vi "Accurate Measure With Setting - 複製 (2).vi"(0 "DMM ref in":refnum<visa-resource-name>, 1 "channel_count":i32=11, 2 "P_current_count":i32, 3 "N_current_count":i32, 5 "DMM error in":errorcluster, 7 "Accurate Measure Setting":T1, 9 "ESP32 ref in":refnum<visa-resource-name>, 11 "ESP32 error in":errorcluster, 12 "current_mode":u8[](array[numeric])=[0, 0, 0, 0, 0, 0, 0, 0, 0, 0, 0]) -> (4 "DMM ref out":refnum<visa-resource-name>, 6 "DMM error out":errorcluster, 8 "Accurate Data":dbl[](array[numeric]), 10 "ESP32 ref out":refnum<visa-resource-name>, 13 "time_out_count":i32, 14 "Standard Deviation of Data":dbl[](array[numeric]), 15 "ESP32 error out":errorcluster)   [LabVIEW 2023]
uses:
  <instrlib>/Agilent 3446X Series/Agilent 3446X Series.lvlib
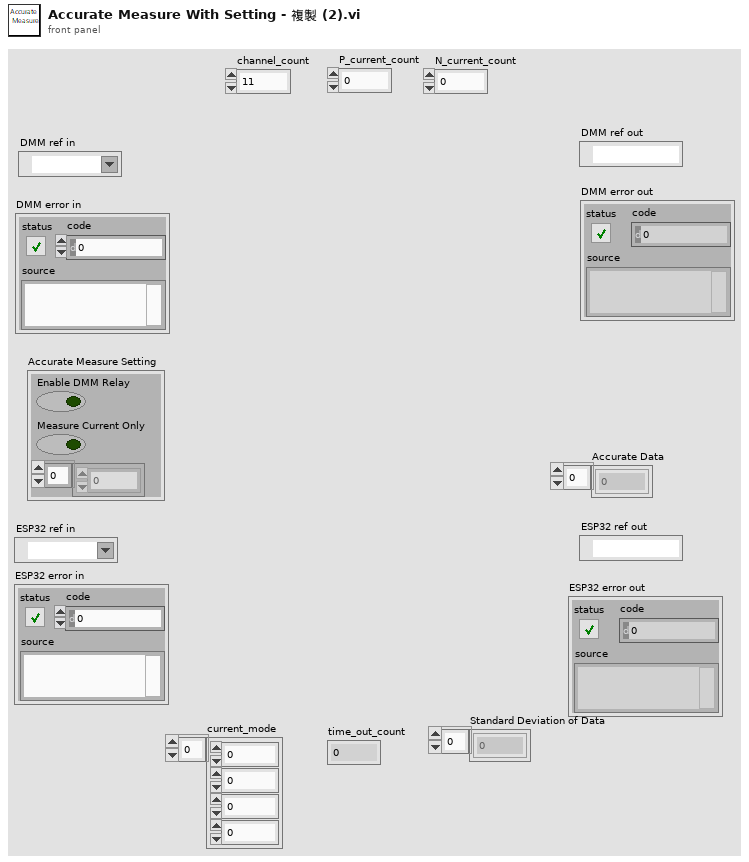
[diagram p1: front panel]
types:
  T1 = cluster{"Enable DMM Relay":bool, "Measure Current Only":bool, dbl[]}
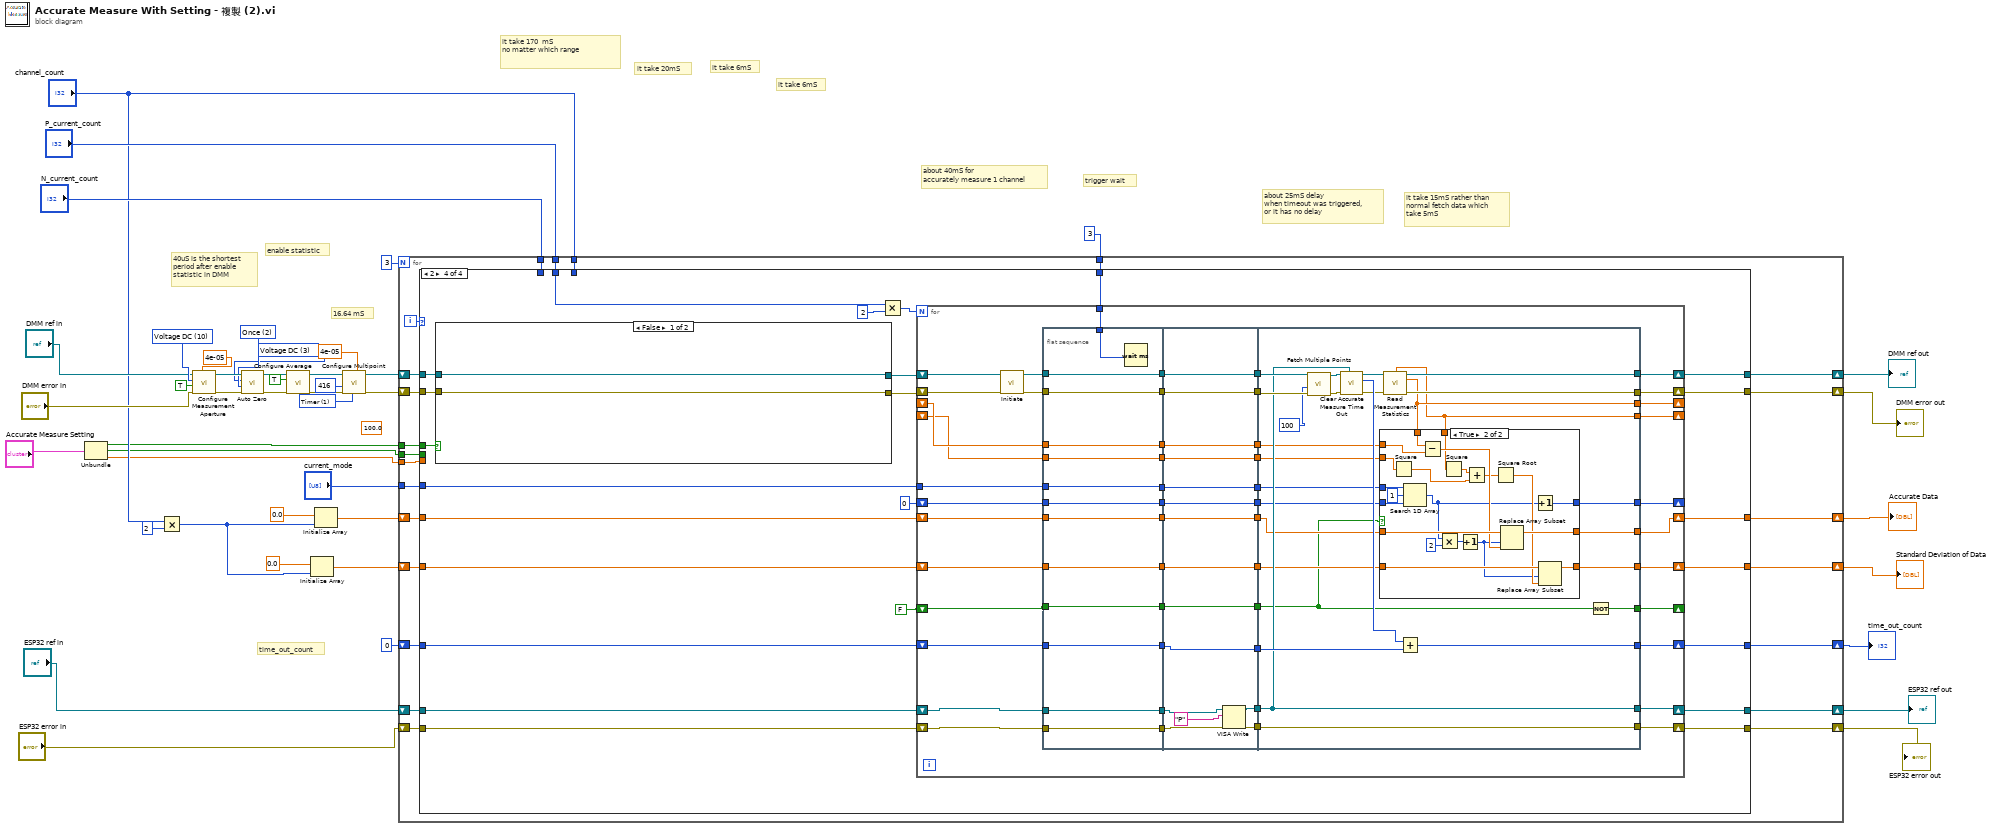
[diagram p0: block diagram]
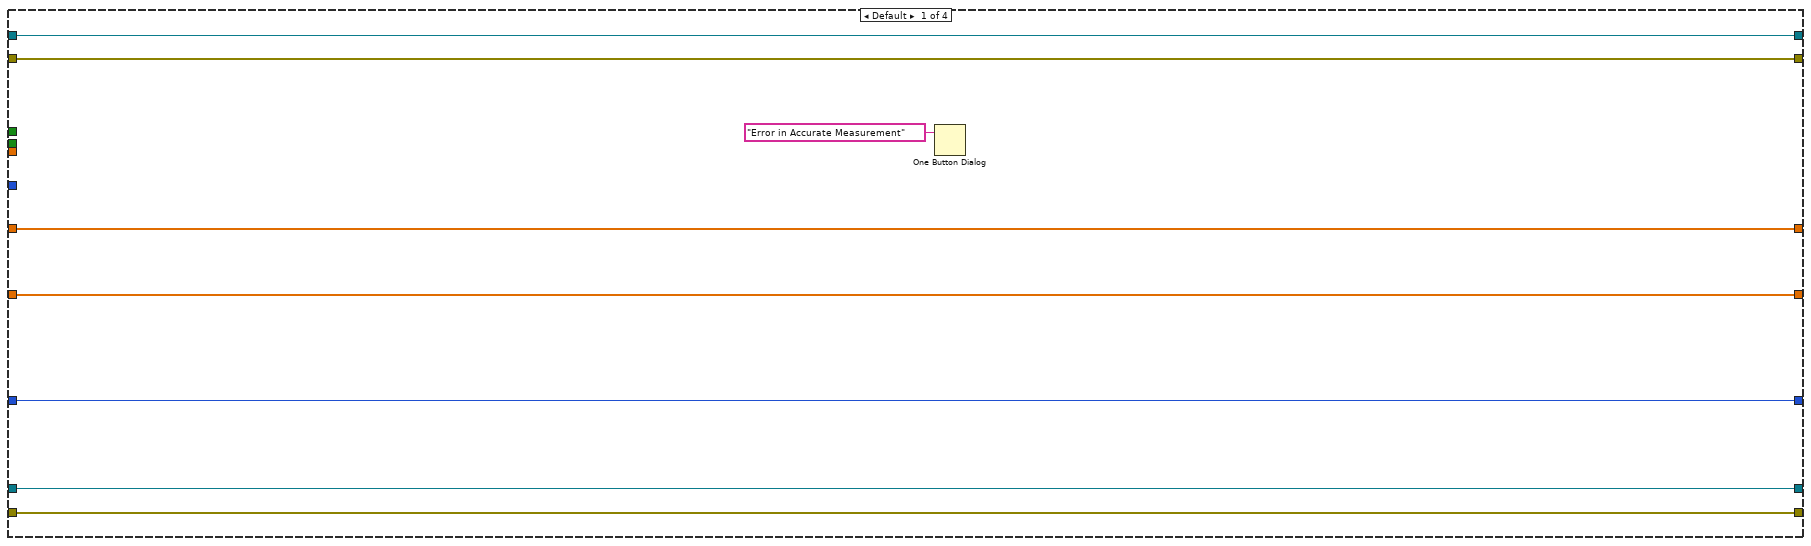
[diagram p2: hidden frame]
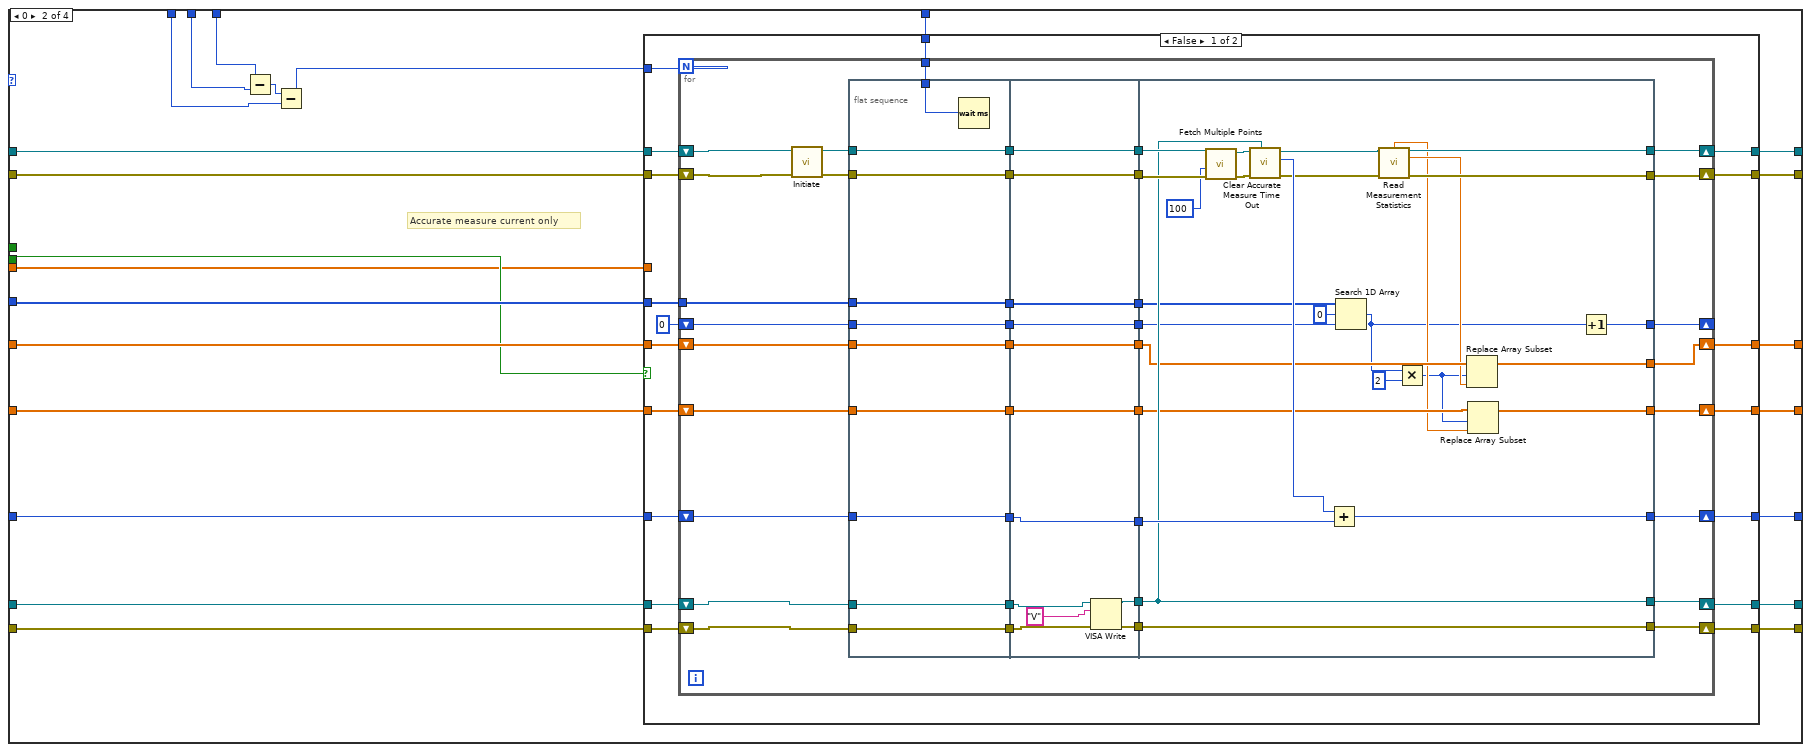
[diagram p3: hidden frame]
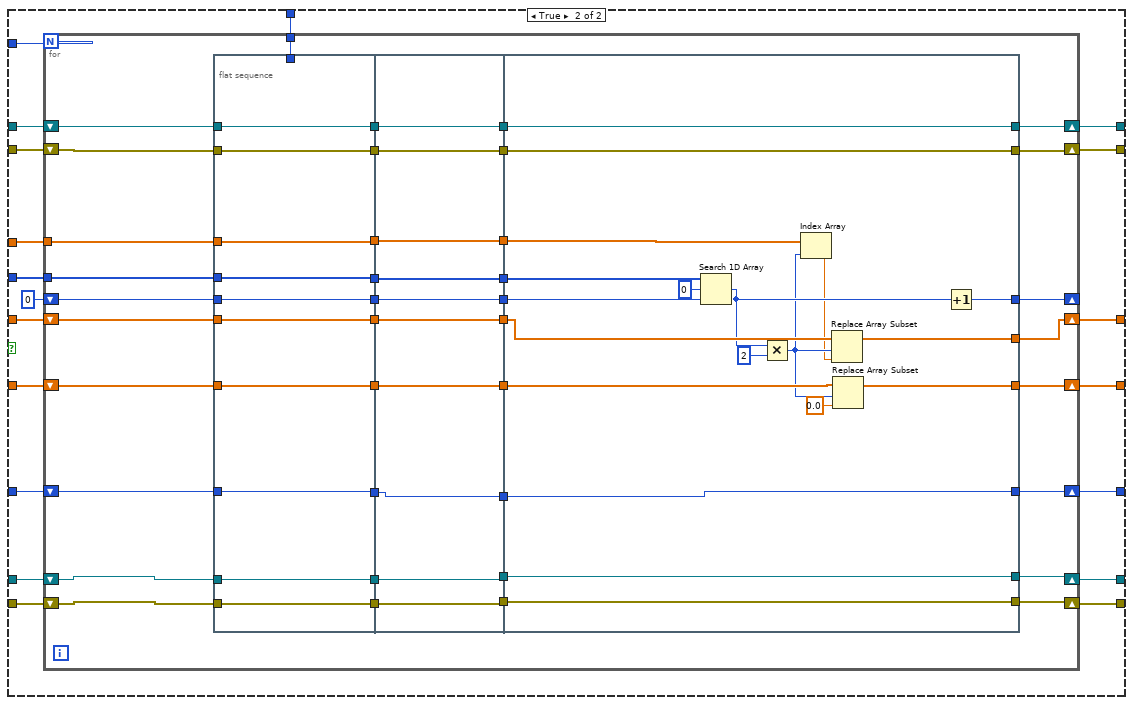
[diagram p4: hidden frame]
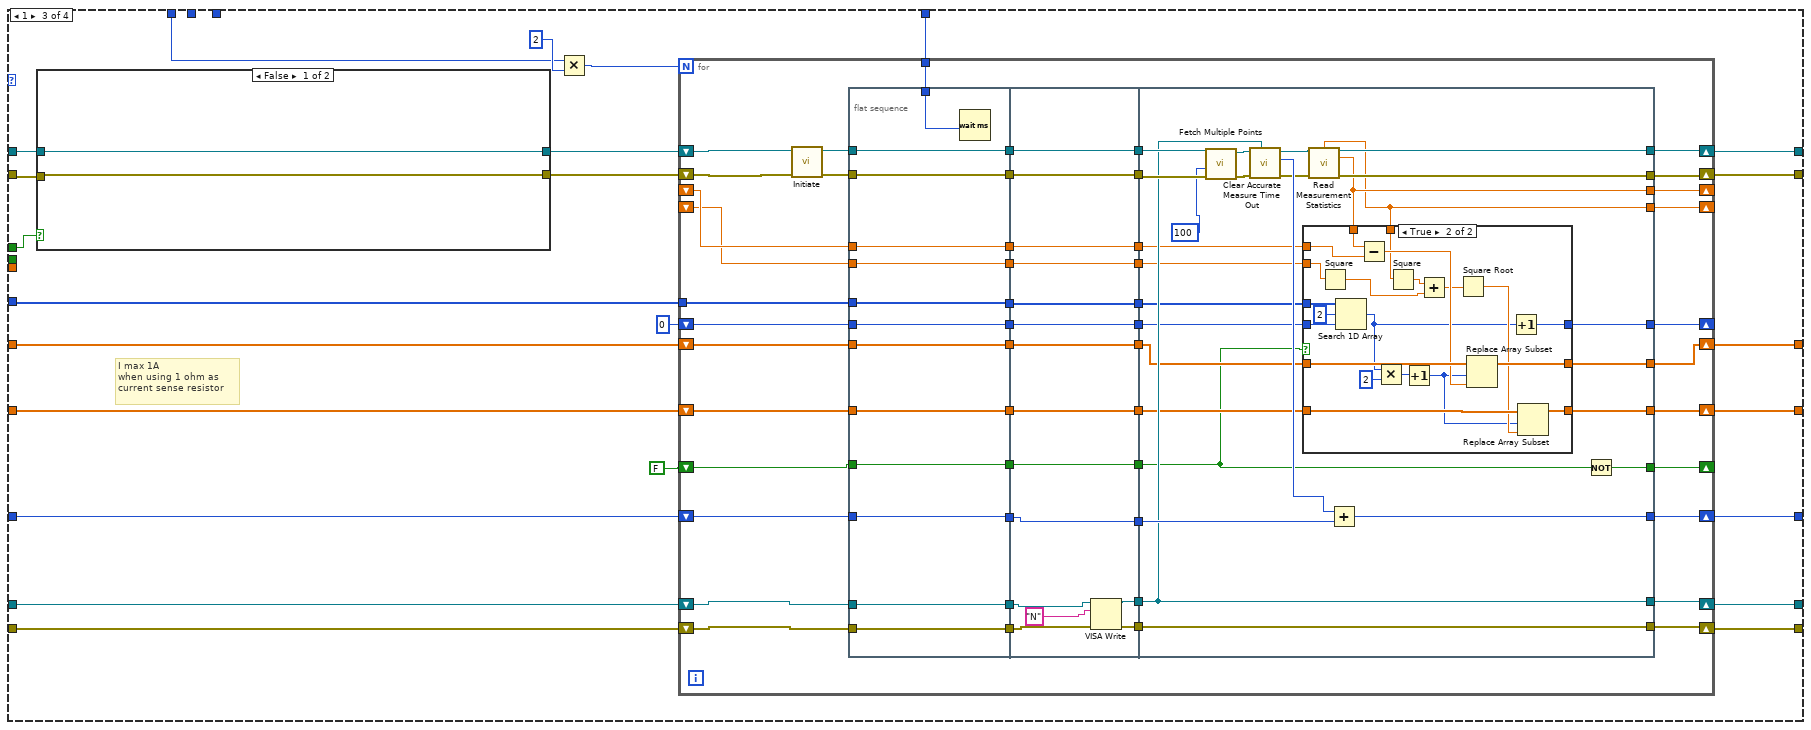
[diagram p5: hidden frame]
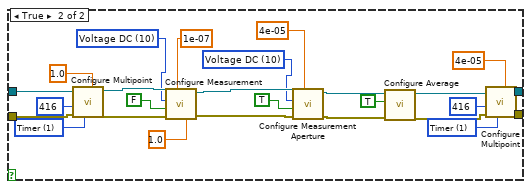
[diagram p6: hidden frame]
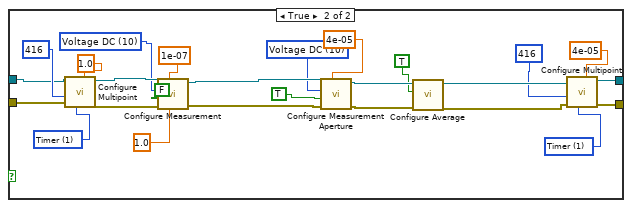
[diagram p8: hidden frame]
diagram:
  (unwired) 100.0 ("Manual Range (1)")
  w32 = 1 items=["Immediate", "Timer"] ("Sample Source (0: Immediate)")
  w39 = 3 items=["Current DC", "Resistance", "Temperature", "Voltage DC"] ("Zero Type (0: Current DC)")
  w40 = 2 items=["Disable", "Enable", "Once"] ("Auto Zero (1: Enable)")
  w36 = 10 items=["Continuity", "Current AC", "Current DC", "Diode", "Frequency", "Resistance 4-wire", "Period", "Resistance 2-wire", "Temperature", "Voltage AC", "Voltage DC", "Voltage DC Ratio", "Capacitance"] ("Measurement Function (0: Continuity)")
  # "it take 6mS"
  # "it take 6mS"
  # "it take 20mS"
  # "it take 170  mS\nno matter which range"
  # "it take 15mS rather than\nnormal fetch data which \ntake 5mS"
  # "about 40mS for \naccurately measure 1 channel"
  # "about 25mS delay\nwhen timeout was triggered,\nor it has no delay"
  # "time_out_count"
  # "trigger wait"
  # "16.64 mS"
  # "enable statistic"
  # "40uS is the shortest\nperiod after enable \nstatistic in DMM"
  n1 = Unbundle("Accurate Measure Setting") -> ("Enable DMM Relay"=w4:bool, "Measure Current Only"=w2:bool, w1:dbl[])
  n2 = Multiply(x="channel_count", y=2) -> (x*y=w5:i32)
  n3 = call <instrlib>:"Configure Measurement Aperture.vi"("Aperture Time (0.1s)"=4e-05, "error in (no error)"="DMM error in", "Enable Aperture (F: Disable)"=TRUE, "Measurement Function (0: Continuity)"=w36, "VISA resource name"="DMM ref in") -> ("error out"=w43:errorcluster, "VISA resource name out"=w42:refnum<visa-resource-name>)  [unwired: 5 in]
  n4 = call <instrlib>:"Auto Zero.vi"("error in (no error)"=w43, "Auto Zero (1: Enable)"=w40, "Zero Type (0: Current DC)"=w39, "VISA resource name"=w42) -> ("error out"=w45:errorcluster, "VISA resource name out"=w44:refnum<visa-resource-name>)  [unwired: 6 in]
  n5 = call <instrlib>:"Configure Average.vi"("error in (no error)"=w45, "Enable Statistics (F: Disable)"=TRUE, "VISA resource name"=w44) -> ("error out"=w34:errorcluster, "VISA resource name out"=w35:refnum<visa-resource-name>)  [unwired: 7 in]
  n6 = Initialize Array(0.0 ("Arithmetic Mean"), w5) -> (w15:dbl[])
  n7 = Initialize Array(0.0 ("Arithmetic Mean"), w5) -> (w18:dbl[])
  n8 = call <instrlib>:"Configure Multipoint.vi"("Sample Interval (1 Second)"=4e-05, "Sample Source (0: Immediate)"=w32, "error in (no error)"=w34, "Sample Count (1)"=416, "VISA resource name"=w35) -> ("error out"=w29:errorcluster, "VISA resource name out"=w30:refnum<visa-resource-name>)  [unwired: 2 in, 3 out]
  n9 = for {
    N: 3 -> [_]
    shift-right: [w66] -> w11
    shift-left: "ESP32 ref in" -> [w68]
    shift-right: [w65] -> w10
    shift-left: "ESP32 error in" -> [w67]
    shift-right: [w62] -> w13
    shift-left: w30 -> [w64]
    shift-right: [w61] -> w12
    shift-left: w29 -> [w63]
    tunnel: "channel_count" -> [w60]
    tunnel: "P_current_count" -> [w59]
    tunnel: "N_current_count" -> [w58]
    tunnel: u32 3 ("milliseconds to wait") -> [w57]
    shift-right: [w56] -> w20
    shift-left: 0 -> [w55]
    shift-right: [w49] -> w9
    shift-left: w18 -> [w54]
    tunnel: "current_mode" -> [w53]
    shift-right: [w50] -> w8
    shift-left: w15 -> [w51]
    tunnel: w4 -> [w48]
    tunnel: w2 -> [w47]
    tunnel: w1 -> [w46]
    i -> [w52]
    n10 = case shown="2" w52 {
      tunnel: w68 -> [w74 w95 w325 w506]
      tunnel: w67 -> [w73 w94 w324 w505]
      tunnel: [w74 w91 w321 w502] -> w66
      tunnel: [w73 w90 w320 w501] -> w65
      tunnel: w64 -> [w76 w97 w309 w489]
      tunnel: w63 -> [w75 w96 w308 w488]
      tunnel: [w76 w93 w323 w504] -> w62
      tunnel: [w75 w92 w322 w503] -> w61
      tunnel: w60 -> [_ w89 _ _]
      tunnel: w59 -> [_ w88 _ w485]
      tunnel: w58 -> [_ w87 w304 _]
      tunnel: [w70 w85 w318 w499] -> w56
      tunnel: w57 -> [_ w86 w319 w500]
      tunnel: w55 -> [w70 w84 w317 w498]
      tunnel: w54 -> [w72 w82 w315 w496]
      tunnel: w53 -> [_ w83 w316 w497]
      tunnel: w51 -> [w71 w81 w313 w494]
      tunnel: [w71 w80 w312 w493] -> w50
      tunnel: [w72 w79 w311 w492] -> w49
      tunnel: w48 -> [_ _ w302 w483]
      tunnel: w47 -> [_ w78 _ _]
      tunnel: w46 -> [_ w77 _ _]
      frame Default {
        n11 = One Button Dialog(message="Error in Accurate Measurement") -> ()  [unwired: 1 in, 1 out]
      }
      frame 0 {
        # "Accurate measure current only"
        n12 = Subtract(x=w89, y=w88) -> (x-y=w99:i32)
        n13 = Subtract(x=w99, y=w87) -> (x-y=w98:i32)
        n14 = case shown="False" w78 {
          tunnel: w98 -> [w117 w223]
          tunnel: w97 -> [w116 w222]
          tunnel: w96 -> [w115 w221]
          tunnel: w95 -> [w114 w220]
          tunnel: w94 -> [w113 w219]
          tunnel: [w112 w218] -> w93
          tunnel: [w111 w217] -> w92
          tunnel: [w110 w216] -> w91
          tunnel: [w109 w215] -> w90
          tunnel: w86 -> [w108 w214]
          tunnel: [w107 w213] -> w85
          tunnel: w84 -> [w106 w212]
          tunnel: w83 -> [w105 w211]
          tunnel: w82 -> [w104 w210]
          tunnel: w81 -> [w102 w208]
          tunnel: [w101 w207] -> w80
          tunnel: [w100 w206] -> w79
          tunnel: w77 -> [_ w205]
          frame False {
            n15 = for {
              N: w117 -> [_]
              shift-right: [w151] -> w112
              shift-left: w116 -> [w155]
              shift-right: [w150] -> w111
              shift-left: w115 -> [w154]
              shift-right: [w149] -> w110
              shift-left: w114 -> [w153]
              shift-right: [w148] -> w109
              shift-left: w113 -> [w152]
              tunnel: w108 -> [w134]
              shift-right: [w133] -> w107
              shift-left: w106 -> [w147]
              tunnel: w105 -> [w131]
              shift-right: [w119] -> w100
              shift-left: w104 -> [w128]
              shift-right: [w123] -> _
              shift-left: 0 ("index of element") -> [w124]
              shift-right: [w118] -> w101
              shift-left: w102 -> [w121]
              n16 = call <instrlib>:"Initiate.vi"("error in (no error)"=w154, "VISA resource name"=w155) -> ("error out"=w135:errorcluster, "VISA resource name out"=w136:refnum<visa-resource-name>)  [unwired: 8 in]
              n17 = flat-sequence {
                tunnel: [w165] -> w146
                tunnel: w153 -> [w165]
                tunnel: [w164] -> w145
                tunnel: w152 -> [w164]
                tunnel: w136 -> [w163]
                tunnel: [w163] -> w144
                tunnel: [w162] -> w143
                tunnel: w135 -> [w162]
                tunnel: [w161] -> w142
                tunnel: w147 -> [w161]
                tunnel: w134 -> [w160]
                tunnel: [w159] -> w132
                tunnel: w131 -> [w159]
                tunnel: [w158] -> w129
                tunnel: w128 -> [w158]
                tunnel: w124 -> [w157]
                tunnel: [w157] -> w126
                tunnel: [w156] -> w122
                tunnel: w121 -> [w156]
                tunnel: w146 -> [w177]
                tunnel: w145 -> [w176]
                tunnel: w144 -> [w175]
                tunnel: [w175] -> w138
                tunnel: w143 -> [w174]
                tunnel: [w174] -> w139
                tunnel: [w173] -> w140
                tunnel: [w172] -> w141
                tunnel: w142 -> [w170]
                tunnel: [w170] -> w137
                tunnel: w132 -> [w169]
                tunnel: [w169] -> w130
                tunnel: w129 -> [w168]
                tunnel: [w168] -> w127
                tunnel: w126 -> [w167]
                tunnel: [w167] -> w125
                tunnel: w122 -> [w166]
                tunnel: [w166] -> w120
                tunnel: [w204] -> w148
                tunnel: [w192] -> w149
                tunnel: [w196] -> w150
                tunnel: [w197] -> w151
                tunnel: w141 -> [w204]
                tunnel: w140 -> [w192]
                tunnel: w139 -> [w203]
                tunnel: w138 -> [w202]
                tunnel: [w198] -> w133
                tunnel: w137 -> [w193]
                tunnel: w130 -> [w191]
                tunnel: w127 -> [w187]
                tunnel: w125 -> [w189]
                tunnel: [w188] -> w123
                tunnel: w120 -> [w185]
                tunnel: [w183] -> w119
                tunnel: [w182] -> w118
                frame #0 {
                  n18 = Wait (ms)(milliseconds to wait=w160) -> ()  [unwired: 1 out]
                }
                frame #1 {
                  n19 = VISA Write(VISA resource name=w177, write buffer="V" ("data in"), error in (no error)=w176) -> (VISA resource name out=w173:refnum<visa-resource-name>, error out=w172:errorcluster)  [unwired: 1 out]
                }
                frame #2 {
                  n20 = call <instrlib>:"Fetch Multiple Points.vi"("error in (no error)"=w203, "Timeout (10000 ms)"=100, "VISA resource name"=w202) -> ("error out"=w200:errorcluster, "VISA resource name out"=w201:refnum<visa-resource-name>)  [unwired: 1 in, 6 out]
                  n21 = call "Clear Accurate Measure Time Out.vi"("ESP32 ref"=w192, "error in (no error)"=w200, "DMM ref"=w201) -> ("error out"=w194:errorcluster, "Time out count"=w199:i32, "VISA Refnum out"=w195:refnum<visa-resource-name>)  [unwired: 5 in, 1 out]
                  n22 = Add(x=w199, y=w193) -> (x+y=w198:i32)
                  n23 = Search 1D Array(1D array=w191, element=u8 0, start index (0)=w189) -> (index of element=w180:i32)
                  n24 = call <instrlib>:"Read Measurement Statistics.vi"("VISA resource name"=w195, "error in (no error)"=w194) -> ("Standard Deviation"=w184:dbl, "VISA resource name out"=w197:refnum<visa-resource-name>, "Arithmetic Mean"=w186:dbl, "error out"=w196:errorcluster)  [unwired: 6 in, 4 out]
                  n25 = Multiply(x=w180, y=2) -> (x*y=w178:i32)
                  n26 = Replace Array Subset(array=w187, new element=w186, index=w178) -> (w183:dbl[])
                  n27 = Replace Array Subset(array=w185, new element=w184, index=w178) -> (w182:dbl[])
                  n28 = Increment(x=w180) -> (x+1=w188:i32)
                }
              }
            }
          }
          frame True {
            n29 = for {
              N: w223 -> [_]
              shift-right: [w232] -> w218
              shift-left: w222 -> [w234]
              shift-right: [w227] -> w217
              shift-left: w221 -> [w229]
              shift-right: [w260] -> w216
              shift-left: w220 -> [w262]
              shift-right: [w259] -> w215
              shift-left: w219 -> [w261]
              tunnel: w214 -> [w251]
              shift-right: [w250] -> w213
              shift-left: w212 -> [w258]
              tunnel: w211 -> [w248]
              shift-right: [w236] -> w206
              shift-left: w210 -> [w245]
              shift-right: [w240] -> _
              shift-left: 0 ("index of element") -> [w241]
              shift-right: [w235] -> w207
              shift-left: w208 -> [w238]
              tunnel: w205 -> [w224]
              n30 = flat-sequence {
                tunnel: [w272] -> w257
                tunnel: w262 -> [w272]
                tunnel: [w271] -> w256
                tunnel: w261 -> [w271]
                tunnel: [w270] -> w255
                tunnel: w258 -> [w270]
                tunnel: w251 -> [_]
                tunnel: [w269] -> w249
                tunnel: w248 -> [w269]
                tunnel: [w268] -> w246
                tunnel: w245 -> [w268]
                tunnel: w241 -> [w267]
                tunnel: [w267] -> w243
                tunnel: [w266] -> w239
                tunnel: w238 -> [w266]
                tunnel: w234 -> [w265]
                tunnel: [w265] -> w231
                tunnel: [w264] -> w230
                tunnel: w229 -> [w264]
                tunnel: [w263] -> w226
                tunnel: w224 -> [w263]
                tunnel: w257 -> [w275]
                tunnel: w256 -> [w274]
                tunnel: [w275] -> w253
                tunnel: [w274] -> w254
                tunnel: w255 -> [w282]
                tunnel: [w282] -> w252
                tunnel: w249 -> [w281]
                tunnel: [w281] -> w247
                tunnel: w246 -> [w280]
                tunnel: [w280] -> w244
                tunnel: w243 -> [w279]
                tunnel: [w279] -> w242
                tunnel: w239 -> [w278]
                tunnel: [w278] -> w237
                tunnel: [w277] -> w233
                tunnel: w231 -> [w277]
                tunnel: w230 -> [w276]
                tunnel: [w276] -> w228
                tunnel: w226 -> [w273]
                tunnel: [w273] -> w225
                tunnel: [w301] -> w259
                tunnel: [w300] -> w260
                tunnel: w254 -> [w301]
                tunnel: w253 -> [w300]
                tunnel: [w283] -> w250
                tunnel: w252 -> [w283]
                tunnel: w247 -> [w299]
                tunnel: w244 -> [w295]
                tunnel: w242 -> [w297]
                tunnel: [w296] -> w240
                tunnel: w237 -> [w294]
                tunnel: [w293] -> w236
                tunnel: [w292] -> w235
                tunnel: w233 -> [w289]
                tunnel: [w289] -> w232
                tunnel: [w288] -> w227
                tunnel: w228 -> [w288]
                tunnel: w225 -> [w286]
                frame #0 {
                }
                frame #1 {
                }
                frame #2 {
                  n31 = Search 1D Array(1D array=w299, element=u8 0, start index (0)=w297) -> (index of element=w291:i32)
                  n32 = Multiply(x=w291, y=2) -> (x*y=w285:i32)
                  n33 = Index Array(array=w286, index=w285) -> (element=w284:dbl)
                  n34 = Replace Array Subset(array=w295, new element=w284, index=w285) -> (w293:dbl[])
                  n35 = Replace Array Subset(array=w294, new element=0.0 ("new element/subarray"), index=w285) -> (w292:dbl[])
                  n36 = Increment(x=w291) -> (x+1=w296:i32)
                }
              }
            }
          }
        }
      }
      frame 1 {
        # "I max 1A\nwhen using 1 ohm as \ncurrent sense resistor"
        n37 = case shown="False" w302 {
          tunnel: w309 -> [w327 w333]
          tunnel: w308 -> [w326 w332]
          tunnel: [w327 w331] -> w307
          tunnel: [w326 w330] -> w306
          frame False {
          }
          frame True {
            w343 = 1 items=["Immediate", "Timer"] ("Sample Source (0: Immediate)")
            w339 = 10 items=["Continuity", "Current AC", "Current DC", "Diode", "Frequency", "Resistance 4-wire", "Period", "Resistance 2-wire", "Temperature", "Voltage AC", "Voltage DC", "Voltage DC Ratio", "Capacitance"] ("Measurement Function (0: Continuity)")
            w337 = 1 items=["Immediate", "Timer"] ("Sample Source (0: Immediate)")
            w334 = 10 items=["Continuity", "Current AC", "Current DC", "Diode", "Frequency", "Resistance 4-wire", "Period", "Resistance 2-wire", "Temperature", "Voltage AC", "Voltage DC", "Voltage DC Ratio", "Capacitance"] ("Measurement Function (10: Voltage DC)")
            n38 = call <instrlib>:"Configure Multipoint.vi"("Sample Interval (1 Second)"=1.0, "Sample Source (0: Immediate)"=w337, "error in (no error)"=w332, "Sample Count (1)"=416, "VISA resource name"=w333) -> ("error out"=w350:errorcluster, "VISA resource name out"=w349:refnum<visa-resource-name>)  [unwired: 2 in, 3 out]
            n39 = call <instrlib>:"Configure Measurement.vi"("Manual Range (1)"=1.0, "Absolute Resolution (1E-6)"=1e-07 ("x"), "error in (no error)"=w350, "Auto Range (T: Enable)"=FALSE, "Measurement Function (10: Voltage DC)"=w334, "VISA resource name"=w349) -> ("error out"=w347:errorcluster, "VISA resource name out"=w348:refnum<visa-resource-name>)  [unwired: 4 out]
            n40 = call <instrlib>:"Configure Measurement Aperture.vi"("Aperture Time (0.1s)"=4e-05, "error in (no error)"=w347, "Enable Aperture (F: Disable)"=TRUE, "Measurement Function (0: Continuity)"=w339, "VISA resource name"=w348) -> ("error out"=w352:errorcluster, "VISA resource name out"=w353:refnum<visa-resource-name>)  [unwired: 5 in]
            n41 = call <instrlib>:"Configure Average.vi"("error in (no error)"=w352, "Enable Statistics (F: Disable)"=TRUE, "VISA resource name"=w353) -> ("error out"=w351:errorcluster, "VISA resource name out"=w346:refnum<visa-resource-name>)  [unwired: 7 in]
            n42 = call <instrlib>:"Configure Multipoint.vi"("Sample Interval (1 Second)"=4e-05, "Sample Source (0: Immediate)"=w343, "error in (no error)"=w351, "Sample Count (1)"=416, "VISA resource name"=w346) -> ("error out"=w330:errorcluster, "VISA resource name out"=w331:refnum<visa-resource-name>)  [unwired: 2 in, 3 out]
          }
        }
        n43 = Multiply(x=w304, y=2) -> (x*y=w305:i32)
        n44 = for {
          N: w305 -> [_]
          shift-right: [w399] -> w323
          shift-left: w307 -> [w403]
          shift-right: [w398] -> w322
          shift-left: w306 -> [w402]
          shift-right: [w397] -> w321
          shift-left: w325 -> [w401]
          shift-right: [w396] -> w320
          shift-left: w324 -> [w400]
          tunnel: w319 -> [w382]
          shift-right: [w381] -> w318
          shift-left: w317 -> [w395]
          tunnel: w316 -> [w379]
          shift-right: [w367] -> w311
          shift-left: w315 -> [w376]
          shift-right: [w371] -> _
          shift-left: 0 ("index of element") -> [w372]
          shift-right: [w366] -> w312
          shift-left: w313 -> [w369]
          shift-right: [w362] -> _
          shift-left: FALSE ("Enable Statistics (F: Disable)") -> [w363]
          shift-right: [w361] -> _
          shift-left: _ -> [w359]
          shift-right: [w360] -> _
          shift-left: _ -> [w356]
          n45 = call <instrlib>:"Initiate.vi"("error in (no error)"=w402, "VISA resource name"=w403) -> ("error out"=w383:errorcluster, "VISA resource name out"=w384:refnum<visa-resource-name>)  [unwired: 8 in]
          n46 = flat-sequence {
            tunnel: [w416] -> w394
            tunnel: w401 -> [w416]
            tunnel: [w415] -> w393
            tunnel: w400 -> [w415]
            tunnel: w384 -> [w414]
            tunnel: [w414] -> w392
            tunnel: [w413] -> w391
            tunnel: w383 -> [w413]
            tunnel: [w412] -> w390
            tunnel: w395 -> [w412]
            tunnel: w382 -> [w411]
            tunnel: [w410] -> w380
            tunnel: w379 -> [w410]
            tunnel: [w409] -> w377
            tunnel: w376 -> [w409]
            tunnel: w372 -> [w408]
            tunnel: [w408] -> w374
            tunnel: [w407] -> w370
            tunnel: w369 -> [w407]
            tunnel: w363 -> [w406]
            tunnel: [w406] -> w365
            tunnel: w359 -> [w405]
            tunnel: [w405] -> w357
            tunnel: w356 -> [w404]
            tunnel: [w404] -> w355
            tunnel: w394 -> [w431]
            tunnel: w393 -> [w430]
            tunnel: w392 -> [w429]
            tunnel: [w429] -> w386
            tunnel: w391 -> [w428]
            tunnel: [w428] -> w387
            tunnel: [w427] -> w388
            tunnel: [w426] -> w389
            tunnel: w390 -> [w424]
            tunnel: [w424] -> w385
            tunnel: w380 -> [w423]
            tunnel: [w423] -> w378
            tunnel: w377 -> [w422]
            tunnel: [w422] -> w375
            tunnel: w374 -> [w421]
            tunnel: [w421] -> w373
            tunnel: w370 -> [w420]
            tunnel: [w420] -> w368
            tunnel: w365 -> [w419]
            tunnel: [w419] -> w364
            tunnel: [w418] -> w358
            tunnel: w357 -> [w418]
            tunnel: w355 -> [w417]
            tunnel: [w417] -> w354
            tunnel: [w458] -> w396
            tunnel: [w446] -> w397
            tunnel: [w450] -> w398
            tunnel: [w451] -> w399
            tunnel: w389 -> [w458]
            tunnel: w388 -> [w446]
            tunnel: w387 -> [w457]
            tunnel: w386 -> [w456]
            tunnel: [w452] -> w381
            tunnel: w385 -> [w447]
            tunnel: w378 -> [w445]
            tunnel: w375 -> [w442]
            tunnel: w373 -> [w444]
            tunnel: [w443] -> w371
            tunnel: w368 -> [w441]
            tunnel: [w440] -> w367
            tunnel: [w439] -> w366
            tunnel: w364 -> [w438]
            tunnel: [w437] -> w362
            tunnel: [w434] -> w361
            tunnel: [w433] -> w360
            tunnel: w358 -> [w436]
            tunnel: w354 -> [w435]
            frame #0 {
              n47 = Wait (ms)(milliseconds to wait=w411) -> ()  [unwired: 1 out]
            }
            frame #1 {
              n48 = VISA Write(VISA resource name=w431, write buffer="N" ("data in"), error in (no error)=w430) -> (VISA resource name out=w427:refnum<visa-resource-name>, error out=w426:errorcluster)  [unwired: 1 out]
            }
            frame #2 {
              n49 = call <instrlib>:"Fetch Multiple Points.vi"("error in (no error)"=w457, "Timeout (10000 ms)"=100, "VISA resource name"=w456) -> ("error out"=w454:errorcluster, "VISA resource name out"=w455:refnum<visa-resource-name>)  [unwired: 1 in, 6 out]
              n50 = call "Clear Accurate Measure Time Out.vi"("ESP32 ref"=w446, "error in (no error)"=w454, "DMM ref"=w455) -> ("error out"=w448:errorcluster, "Time out count"=w453:i32, "VISA Refnum out"=w449:refnum<visa-resource-name>)  [unwired: 5 in, 1 out]
              n51 = call <instrlib>:"Read Measurement Statistics.vi"("VISA resource name"=w449, "error in (no error)"=w448) -> ("Standard Deviation"=w433:dbl, "VISA resource name out"=w451:refnum<visa-resource-name>, "Arithmetic Mean"=w434:dbl, "error out"=w450:errorcluster)  [unwired: 6 in, 4 out]
              n52 = case shown="True" w438 {
                tunnel: w445 -> [_ w482]
                tunnel: w444 -> [w461 w480]
                tunnel: [w461 w479] -> w443
                tunnel: w442 -> [w460 w478]
                tunnel: w441 -> [w459 w477]
                tunnel: [w460 w476] -> w440
                tunnel: [w459 w475] -> w439
                tunnel: w436 -> [_ w466]
                tunnel: w435 -> [_ w473]
                tunnel: w434 -> [_ w467]
                tunnel: w433 -> [_ w472]
                frame False {
                }
                frame True {
                  n53 = Square(x=w473) -> (x^2=w470:dbl)
                  n54 = Search 1D Array(1D array=w482, element=u8 2, start index (0)=w480) -> (index of element=w463:i32)
                  n55 = Subtract(x=w467, y=w466) -> (x-y=w474:dbl)
                  n56 = Multiply(x=w463, y=2) -> (x*y=w464:i32)
                  n57 = Square(x=w472) -> (x^2=w471:dbl)
                  n58 = Increment(x=w464) -> (x+1=w462:i32)
                  n59 = Add(x=w471, y=w470) -> (x+y=w469:dbl)
                  n60 = Square Root(x=w469) -> (sqrt(x)=w468:dbl)
                  n61 = Replace Array Subset(array=w478, new element=w474, index=w462) -> (w476:dbl[])
                  n62 = Increment(x=w463) -> (x+1=w479:i32)
                  n63 = Replace Array Subset(array=w477, new element=w468, index=w462) -> (w475:dbl[])
                }
              }
              n64 = Add(x=w453, y=w447) -> (x+y=w452:i32)
              n65 = Not(x=w438) -> (.not. x?=w437:bool)
            }
          }
        }
      }
      frame 2 {
        n66 = case shown="False" w483 {
          tunnel: w489 -> [w508 w514]
          tunnel: w488 -> [w507 w513]
          tunnel: [w508 w512] -> w487
          tunnel: [w507 w511] -> w486
          frame False {
          }
          frame True {
            w524 = 1 items=["Immediate", "Timer"] ("Sample Source (0: Immediate)")
            w520 = 10 items=["Continuity", "Current AC", "Current DC", "Diode", "Frequency", "Resistance 4-wire", "Period", "Resistance 2-wire", "Temperature", "Voltage AC", "Voltage DC", "Voltage DC Ratio", "Capacitance"] ("Measurement Function (0: Continuity)")
            w518 = 1 items=["Immediate", "Timer"] ("Sample Source (0: Immediate)")
            w515 = 10 items=["Continuity", "Current AC", "Current DC", "Diode", "Frequency", "Resistance 4-wire", "Period", "Resistance 2-wire", "Temperature", "Voltage AC", "Voltage DC", "Voltage DC Ratio", "Capacitance"] ("Measurement Function (10: Voltage DC)")
            n67 = call <instrlib>:"Configure Multipoint.vi"("Sample Interval (1 Second)"=1.0, "Sample Source (0: Immediate)"=w518, "error in (no error)"=w513, "Sample Count (1)"=416, "VISA resource name"=w514) -> ("error out"=w531:errorcluster, "VISA resource name out"=w530:refnum<visa-resource-name>)  [unwired: 2 in, 3 out]
            n68 = call <instrlib>:"Configure Measurement.vi"("Manual Range (1)"=1.0, "Absolute Resolution (1E-6)"=1e-07 ("x"), "error in (no error)"=w531, "Auto Range (T: Enable)"=FALSE, "Measurement Function (10: Voltage DC)"=w515, "VISA resource name"=w530) -> ("error out"=w528:errorcluster, "VISA resource name out"=w529:refnum<visa-resource-name>)  [unwired: 4 out]
            n69 = call <instrlib>:"Configure Measurement Aperture.vi"("Aperture Time (0.1s)"=4e-05, "error in (no error)"=w528, "Enable Aperture (F: Disable)"=TRUE, "Measurement Function (0: Continuity)"=w520, "VISA resource name"=w529) -> ("error out"=w533:errorcluster, "VISA resource name out"=w534:refnum<visa-resource-name>)  [unwired: 5 in]
            n70 = call <instrlib>:"Configure Average.vi"("error in (no error)"=w533, "Enable Statistics (F: Disable)"=TRUE, "VISA resource name"=w534) -> ("error out"=w532:errorcluster, "VISA resource name out"=w527:refnum<visa-resource-name>)  [unwired: 7 in]
            n71 = call <instrlib>:"Configure Multipoint.vi"("Sample Interval (1 Second)"=4e-05, "Sample Source (0: Immediate)"=w524, "error in (no error)"=w532, "Sample Count (1)"=416, "VISA resource name"=w527) -> ("error out"=w511:errorcluster, "VISA resource name out"=w512:refnum<visa-resource-name>)  [unwired: 2 in, 3 out]
          }
        }
        n72 = Multiply(x=w485, y=2) -> (x*y=w484:i32)
        n73 = for {
          N: w484 -> [_]
          shift-right: [w580] -> w504
          shift-left: w487 -> [w584]
          shift-right: [w579] -> w503
          shift-left: w486 -> [w583]
          shift-right: [w578] -> w502
          shift-left: w506 -> [w582]
          shift-right: [w577] -> w501
          shift-left: w505 -> [w581]
          tunnel: w500 -> [w563]
          shift-right: [w562] -> w499
          shift-left: w498 -> [w576]
          tunnel: w497 -> [w560]
          shift-right: [w548] -> w492
          shift-left: w496 -> [w557]
          shift-right: [w552] -> _
          shift-left: 0 ("index of element") -> [w553]
          shift-right: [w547] -> w493
          shift-left: w494 -> [w550]
          shift-right: [w543] -> _
          shift-left: FALSE ("Enable Statistics (F: Disable)") -> [w544]
          shift-right: [w542] -> _
          shift-left: _ -> [w540]
          shift-right: [w541] -> _
          shift-left: _ -> [w537]
          n74 = call <instrlib>:"Initiate.vi"("error in (no error)"=w583, "VISA resource name"=w584) -> ("error out"=w564:errorcluster, "VISA resource name out"=w565:refnum<visa-resource-name>)  [unwired: 8 in]
          n75 = flat-sequence {
            tunnel: [w597] -> w575
            tunnel: w582 -> [w597]
            tunnel: [w596] -> w574
            tunnel: w581 -> [w596]
            tunnel: w565 -> [w595]
            tunnel: [w595] -> w573
            tunnel: [w594] -> w572
            tunnel: w564 -> [w594]
            tunnel: [w593] -> w571
            tunnel: w576 -> [w593]
            tunnel: w563 -> [w592]
            tunnel: [w591] -> w561
            tunnel: w560 -> [w591]
            tunnel: [w590] -> w558
            tunnel: w557 -> [w590]
            tunnel: w553 -> [w589]
            tunnel: [w589] -> w555
            tunnel: [w588] -> w551
            tunnel: w550 -> [w588]
            tunnel: w544 -> [w587]
            tunnel: [w587] -> w546
            tunnel: w540 -> [w586]
            tunnel: [w586] -> w538
            tunnel: w537 -> [w585]
            tunnel: [w585] -> w536
            tunnel: w575 -> [w612]
            tunnel: w574 -> [w611]
            tunnel: w573 -> [w610]
            tunnel: [w610] -> w567
            tunnel: w572 -> [w609]
            tunnel: [w609] -> w568
            tunnel: [w608] -> w569
            tunnel: [w607] -> w570
            tunnel: w571 -> [w605]
            tunnel: [w605] -> w566
            tunnel: w561 -> [w604]
            tunnel: [w604] -> w559
            tunnel: w558 -> [w603]
            tunnel: [w603] -> w556
            tunnel: w555 -> [w602]
            tunnel: [w602] -> w554
            tunnel: w551 -> [w601]
            tunnel: [w601] -> w549
            tunnel: w546 -> [w600]
            tunnel: [w600] -> w545
            tunnel: [w599] -> w539
            tunnel: w538 -> [w599]
            tunnel: w536 -> [w598]
            tunnel: [w598] -> w535
            tunnel: [w639] -> w577
            tunnel: [w627] -> w578
            tunnel: [w631] -> w579
            tunnel: [w632] -> w580
            tunnel: w570 -> [w639]
            tunnel: w569 -> [w627]
            tunnel: w568 -> [w638]
            tunnel: w567 -> [w637]
            tunnel: [w633] -> w562
            tunnel: w566 -> [w628]
            tunnel: w559 -> [w626]
            tunnel: w556 -> [w623]
            tunnel: w554 -> [w625]
            tunnel: [w624] -> w552
            tunnel: w549 -> [w622]
            tunnel: [w621] -> w548
            tunnel: [w620] -> w547
            tunnel: w545 -> [w619]
            tunnel: [w618] -> w543
            tunnel: [w615] -> w542
            tunnel: [w614] -> w541
            tunnel: w539 -> [w617]
            tunnel: w535 -> [w616]
            frame #0 {
              n76 = Wait (ms)(milliseconds to wait=w592) -> ()  [unwired: 1 out]
            }
            frame #1 {
              n77 = VISA Write(VISA resource name=w612, write buffer="P" ("data in"), error in (no error)=w611) -> (VISA resource name out=w608:refnum<visa-resource-name>, error out=w607:errorcluster)  [unwired: 1 out]
            }
            frame #2 {
              n78 = call <instrlib>:"Fetch Multiple Points.vi"("error in (no error)"=w638, "Timeout (10000 ms)"=100, "VISA resource name"=w637) -> ("error out"=w635:errorcluster, "VISA resource name out"=w636:refnum<visa-resource-name>)  [unwired: 1 in, 6 out]
              n79 = call "Clear Accurate Measure Time Out.vi"("ESP32 ref"=w627, "error in (no error)"=w635, "DMM ref"=w636) -> ("error out"=w629:errorcluster, "Time out count"=w634:i32, "VISA Refnum out"=w630:refnum<visa-resource-name>)  [unwired: 5 in, 1 out]
              n80 = call <instrlib>:"Read Measurement Statistics.vi"("VISA resource name"=w630, "error in (no error)"=w629) -> ("Standard Deviation"=w614:dbl, "VISA resource name out"=w632:refnum<visa-resource-name>, "Arithmetic Mean"=w615:dbl, "error out"=w631:errorcluster)  [unwired: 6 in, 4 out]
              n81 = case shown="True" w619 {
                tunnel: w626 -> [_ w663]
                tunnel: w625 -> [w642 w661]
                tunnel: [w642 w660] -> w624
                tunnel: w623 -> [w641 w659]
                tunnel: w622 -> [w640 w658]
                tunnel: [w641 w657] -> w621
                tunnel: [w640 w656] -> w620
                tunnel: w617 -> [_ w647]
                tunnel: w616 -> [_ w654]
                tunnel: w615 -> [_ w648]
                tunnel: w614 -> [_ w653]
                frame False {
                }
                frame True {
                  n82 = Square(x=w654) -> (x^2=w651:dbl)
                  n83 = Search 1D Array(1D array=w663, element=u8 1, start index (0)=w661) -> (index of element=w644:i32)
                  n84 = Subtract(x=w648, y=w647) -> (x-y=w655:dbl)
                  n85 = Multiply(x=w644, y=2) -> (x*y=w645:i32)
                  n86 = Square(x=w653) -> (x^2=w652:dbl)
                  n87 = Increment(x=w645) -> (x+1=w643:i32)
                  n88 = Add(x=w652, y=w651) -> (x+y=w650:dbl)
                  n89 = Square Root(x=w650) -> (sqrt(x)=w649:dbl)
                  n90 = Replace Array Subset(array=w659, new element=w655, index=w643) -> (w657:dbl[])
                  n91 = Increment(x=w644) -> (x+1=w660:i32)
                  n92 = Replace Array Subset(array=w658, new element=w649, index=w643) -> (w656:dbl[])
                }
              }
              n93 = Add(x=w634, y=w628) -> (x+y=w633:i32)
              n94 = Not(x=w619) -> (.not. x?=w618:bool)
            }
          }
        }
      }
    }
  }
  "time_out_count" <- w20
  "DMM ref out" <- w13
  "DMM error out" <- w12
  "ESP32 ref out" <- w11
  "ESP32 error out" <- w10
  "Accurate Data" <- w9
  "Standard Deviation of Data" <- w8
